vi "XML_getNextTag.vi"(9 "Tag":string, 11 "XML in":string) -> (0 "Value":string, 1 "after Tag":string, 2 "Tag Found":string, 3 "before Tag":string)   [LabVIEW 2012]
doc: "Gets the value of the specified Tag. Supports nested tags. If no Tag is specified, this will return the value of the first tag it finds."
uses:
  <vilib>/regexp/Match Regular Expression.xnode
panel:
  # "<value><array><data>\n    <value>testing</value>\n     <value><boolean>1</boolean></value>\n</data></array></value>"
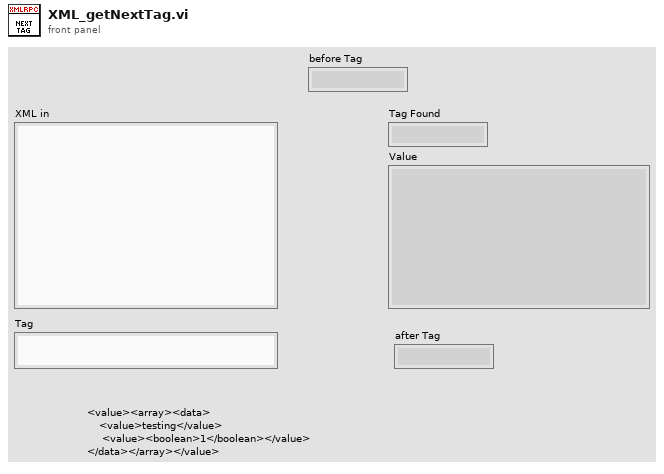
[diagram p1: front panel]
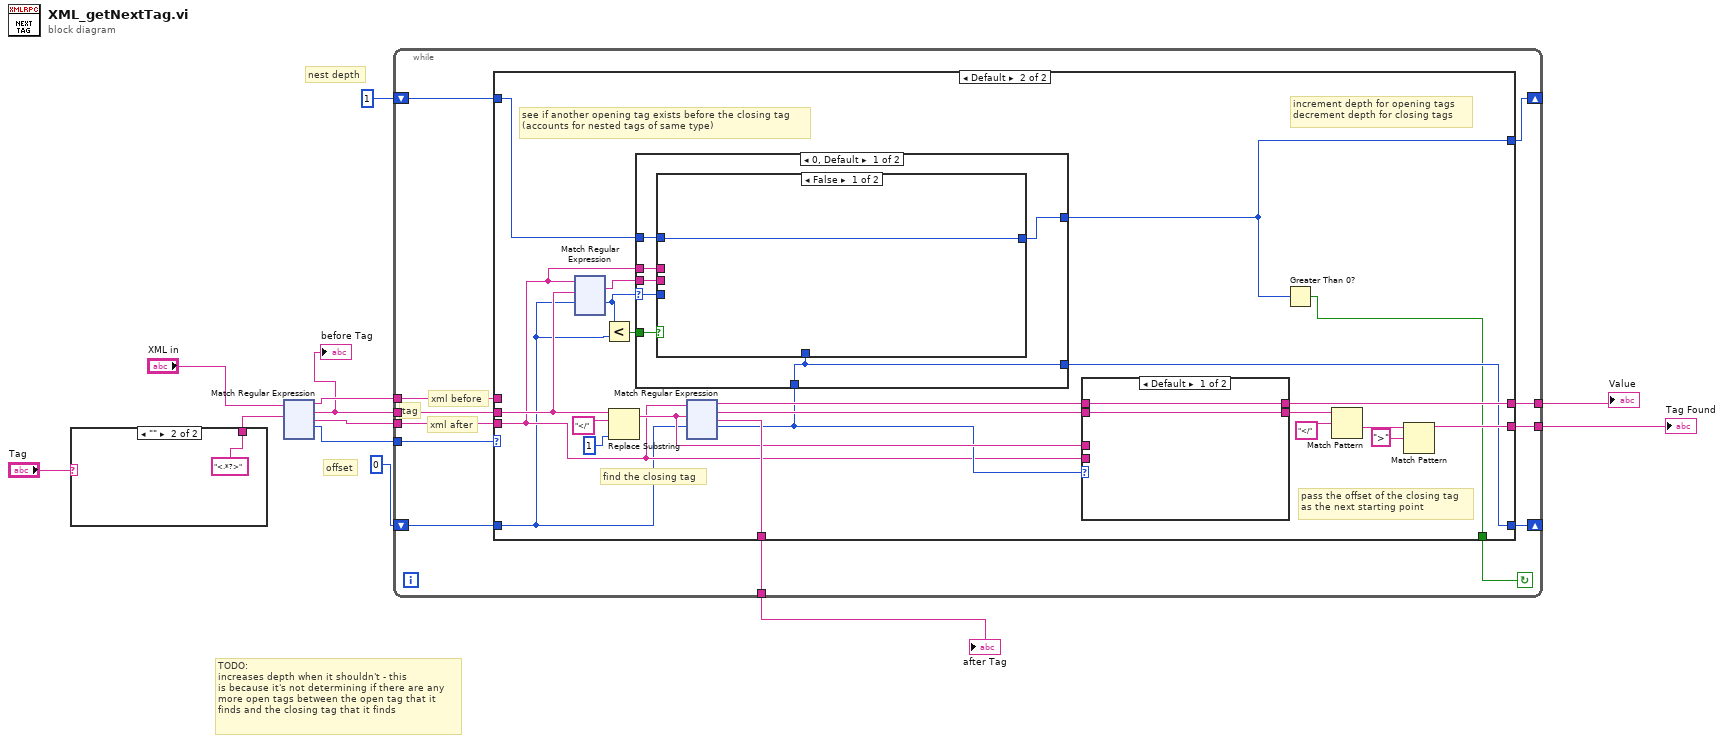
[diagram p0: block diagram]
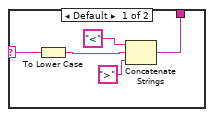
[diagram p2: hidden frame]
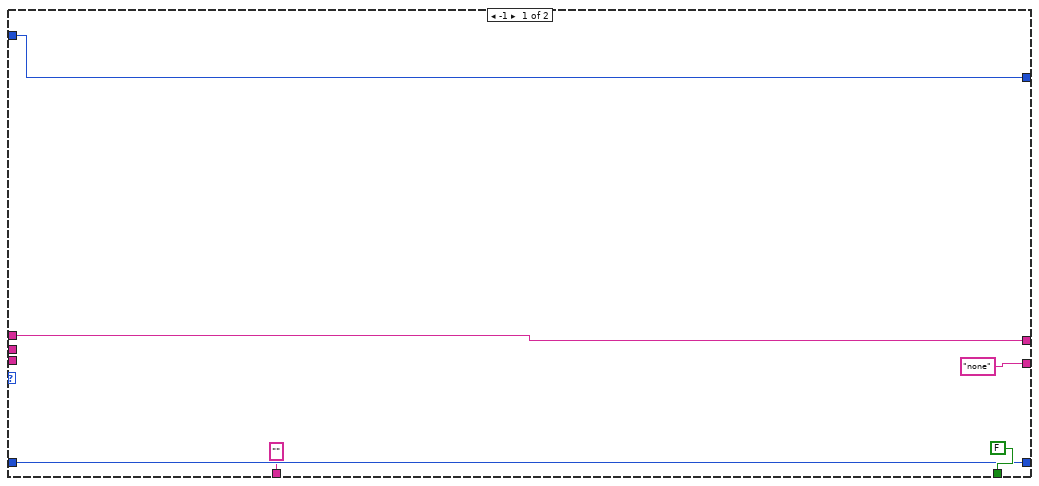
[diagram p3: hidden frame]
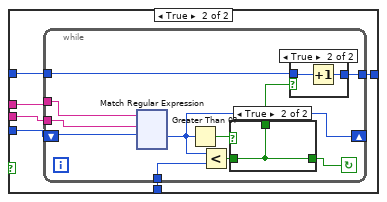
[diagram p4: hidden frame]
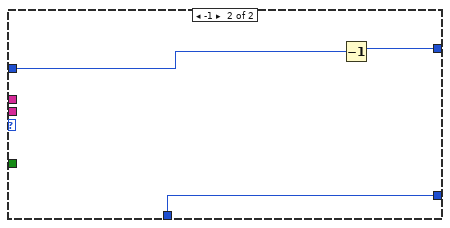
[diagram p7: hidden frame]
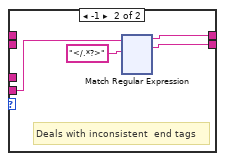
[diagram p8: hidden frame]
diagram:
  # "TODO:\nincreases depth when it shouldn't - this\nis because it's not determining if there are any\nmore open tags between the open tag that it\nfinds and the closing tag that it finds"
  # "nest depth"
  # "offset"
  n1 = case shown="\"\"" "Tag" {
    selector: "Tag" -> [w15 _]
    tunnel: [w13 "<.*?>" ("regular expression")] -> w12
    frame Default {
      n2 = To Lower Case(string=w15) -> (all lower case string=w14:string)
      n3 = Concatenate Strings("<" ("string"), w14, ">" ("string")) -> (w13:string)
    }
    frame "" {
    }
  }
  n4 = xnode "Match Regular Expression"("input string"="XML in", "regular expression"=w12) -> ("before match"=w10:string, "whole match"=w1:string, "after match"=w9:string, "offset past match"=w8:i32)  [unwired: 4 in, 1 out]
  "before Tag" <- w1
  n5 = while {
    tunnel: w10 -> [w30]
    tunnel: w1 -> [w29]
    tunnel: w9 -> [w28]
    tunnel: w8 -> [w27]
    tunnel: [w26] -> w7
    tunnel: [w25] -> w6
    shift-right: [w22] -> _
    shift-left: 0 ("length (len. of substring)") -> [w23]
    shift-right: [w20] -> _
    shift-left: 1 ("length (len. of substring)") -> [w21]
    tunnel: [w19] -> w3
    stop <- w24 continue-if-true
    # "xml before"
    # "xml after"
    # "tag"
    n6 = case shown="Default" w27 {
      tunnel: w28 -> [_ w42]
      tunnel: [w35 w53] -> w25
      tunnel: ["none" ("whole match") w56] -> w26
      tunnel: w30 -> [w35 _]
      tunnel: w29 -> [_ w49]
      tunnel: [FALSE w41] -> w24
      tunnel: w23 -> [w33 w38]
      tunnel: [w33 w45] -> w22
      tunnel: w21 -> [w32 w43]
      tunnel: [w32 w40] -> w20
      tunnel: ["" ("after match") w48] -> w19
      frame -1 {
      }
      frame Default {
        # "pass the offset of the closing tag\nas the next starting point"
        # "increment depth for opening tags\ndecrement depth for closing tags"
        # "see if another opening tag exists before the closing tag\n(accounts for nested tags of same type)"
        # "find the closing tag"
        n7 = xnode "Match Regular Expression"("input string"=w42, "regular expression"=w49, "offset (0)"=w38) -> ("whole match"=w44:string, "offset past match"=w39:i32)  [unwired: 3 in, 3 out]
        n8 = Less?(x=w39, y=w38) -> (x < y?=w37:bool)
        n9 = Replace Substring(2:1 ("length (len. of substring)"), 4:"</" ("substring (\"\")"), 5:w49) -> (1:w47:string)  [unwired: 1 in, 1 out]
        n10 = xnode "Match Regular Expression"("input string"=w42, "regular expression"=w47, "offset (0)"=w38) -> ("before match"=w51:string, "whole match"=w50:string, "after match"=w48:string, "offset past match"=w46:i32)  [unwired: 3 in, 1 out]
        n11 = case shown="0, Default" w39 {
          selector: w39 -> [w62 _]
          tunnel: w46 -> [w61 w203]
          tunnel: [w61 w203] -> w45
          tunnel: w44 -> [w64 _]
          tunnel: w43 -> [w63 w201]
          tunnel: [w66 w202] -> w40
          tunnel: w42 -> [w65 _]
          tunnel: w37 -> [w60 _]
          frame 0, Default {
            n12 = case shown="False" w60 {
              tunnel: [w67 w73] -> w66
              tunnel: w65 -> [_ w72]
              tunnel: w64 -> [_ w71]
              tunnel: w63 -> [w67 w70]
              tunnel: w62 -> [_ w69]
              tunnel: w61 -> [_ w68]
              frame False {
              }
              frame True {
                n13 = while {
                  tunnel: [w84] -> w73
                  tunnel: w70 -> [w78]
                  tunnel: w68 -> [w82]
                  shift-right: [w81] -> _
                  shift-left: w69 -> [w83]
                  tunnel: w72 -> [w80]
                  tunnel: w71 -> [w79]
                  stop <- w75 continue-if-true
                  n14 = xnode "Match Regular Expression"("input string"=w80, "regular expression"=w79, "offset (0)"=w83) -> ("offset past match"=w81:i32)  [unwired: 3 in, 4 out]
                  n15 = Greater Than 0?(x=w81) -> (x > 0?=w77:bool)
                  n16 = Less?(x=w81, y=w82) -> (x < y?=w76:bool)
                  n17 = case shown="True" w77 {
                    selector: w77 -> [w85 _]
                    tunnel: w76 -> [_ w86]
                    tunnel: [w85 w86] -> w75
                    tunnel: [w85 w86] -> w74
                    frame False {
                    }
                    frame True {
                    }
                  }
                  n18 = case shown="True" w74 {
                    tunnel: w78 -> [w87 w89]
                    tunnel: [w87 w88] -> w84
                    frame False {
                    }
                    frame True {
                      n19 = Increment(x=w89) -> (x+1=w88:i32)
                    }
                  }
                }
              }
            }
          }
          frame -1 {
            n20 = Decrement(x=w201) -> (x-1=w202:i32)
          }
        }
        n21 = case shown="Default" w46 {
          tunnel: w42 -> [_ w320]
          tunnel: [w316 w318] -> w53
          tunnel: [w315 w317] -> w52
          tunnel: w51 -> [w316 _]
          tunnel: w50 -> [w315 _]
          tunnel: w47 -> [_ _]
          frame Default {
          }
          frame -1 {
            # "Deals with inconsistent  end tags"
            n22 = xnode "Match Regular Expression"("input string"=w320, "regular expression"="</.*?>") -> ("before match"=w318:string, "whole match"=w317:string)  [unwired: 4 in, 3 out]
          }
        }
        n23 = Greater Than 0?(x=w40) -> (x > 0?=w41:bool)
        n24 = Match Pattern(string=w52, regular expression="</") -> (after substring=w58:string)  [unwired: 1 in, 3 out]
        n25 = Match Pattern(string=w58, regular expression=">") -> (before substring=w56:string)  [unwired: 1 in, 3 out]
      }
    }
  }
  "Tag Found" <- w7
  "Value" <- w6
  "after Tag" <- w3
